vi "change CAD coordinates.vi"() -> ()   [LabVIEW 2020]
uses:
  <vilib>/Analysis/NI_AALPro.lvlib
  <vilib>/Analysis/coordinate.llb/2D Cartesian Coordinate Rotation (Scalar).vi
panel:
  in  "Save to txt file":bool
  in  "Save picture":bool
  out "2D Picture":picture
  in  "Add delamination dots":bool
  out "Array":dbl[][](array[numeric])
  in  "stop":bool
  in  "Rotate by angle":bool
  in  "theta (degrees)":dbl
  in  "Flip Y sign":bool
  in  "Flip X sign":bool
  in  "increase radius":bool
  in  "inc":dbl format="%#_13g"
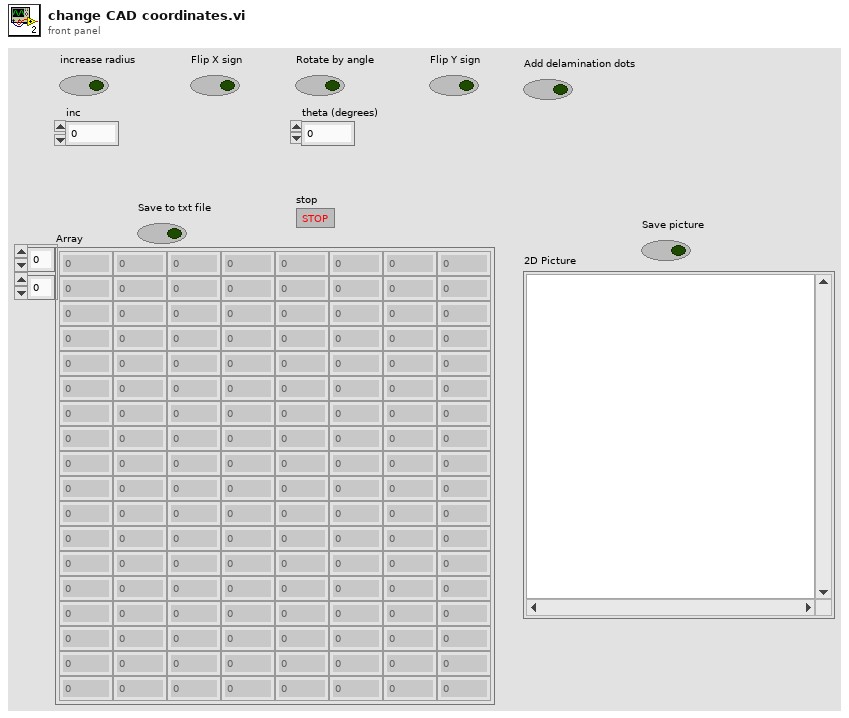
[diagram p1: front panel]
types:
  T1 = typedef "imagedata.ctl" = cluster{"image type":i32, "image depth":i32, "image":u8[], "mask":u8[], "colors":u32[], "Rectangle":cluster{"left":i16, "top":i16, "right":i16, "bottom":i16}}
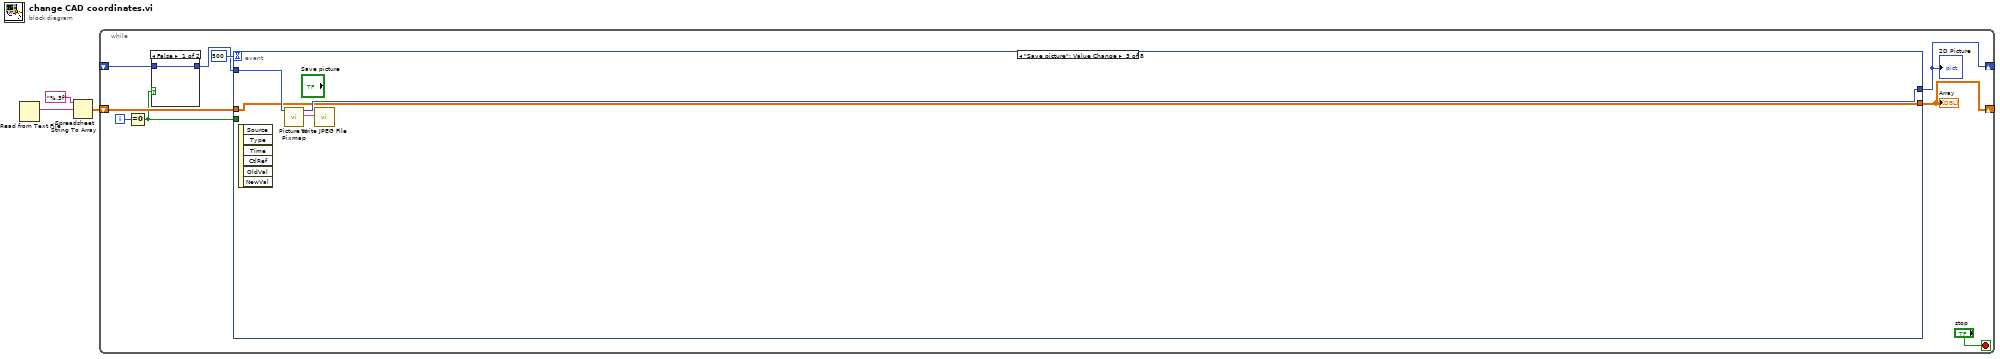
[diagram p0: block diagram]
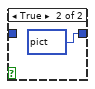
[diagram p2: hidden frame]
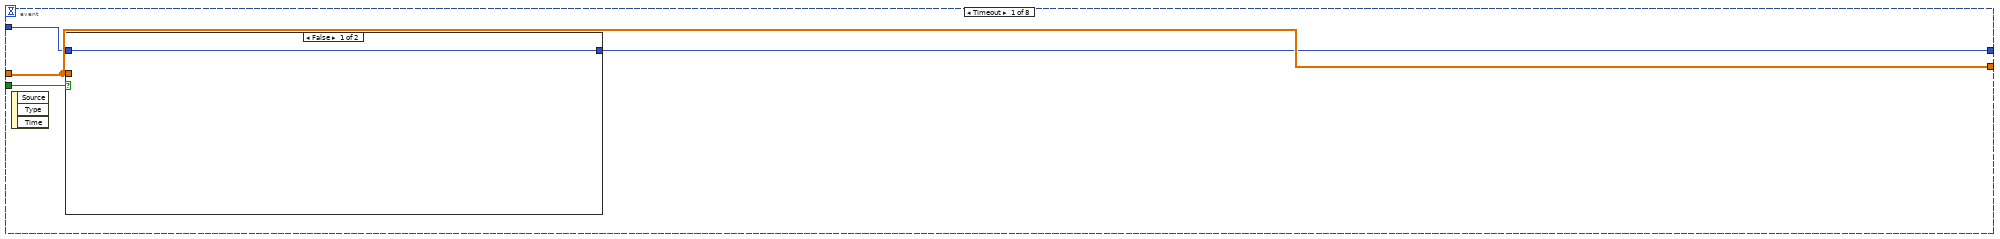
[diagram p3: hidden frame]
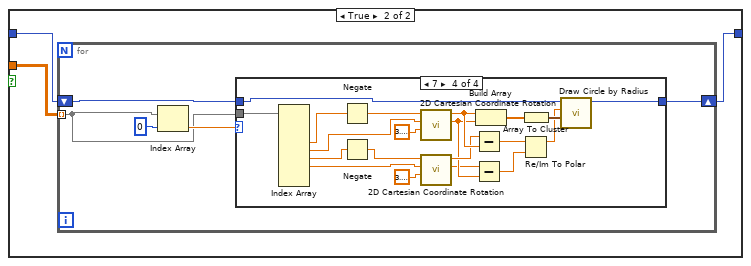
[diagram p4: hidden frame]
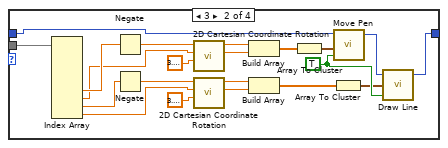
[diagram p6: hidden frame]
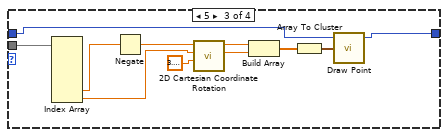
[diagram p7: hidden frame]
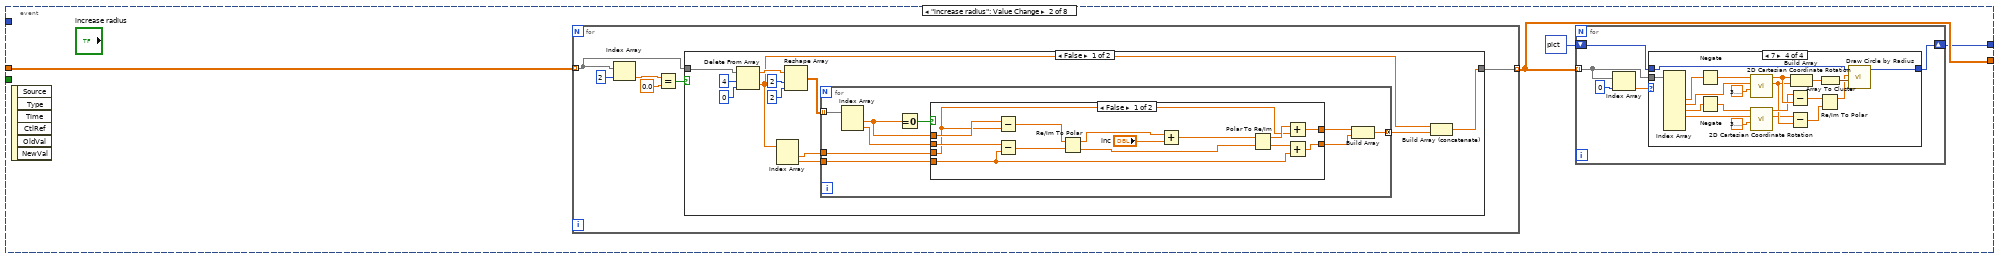
[diagram p8: hidden frame]
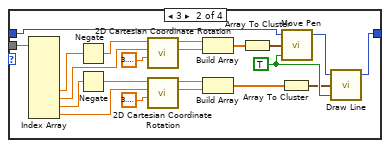
[diagram p10: hidden frame]
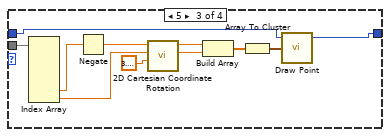
[diagram p11: hidden frame]
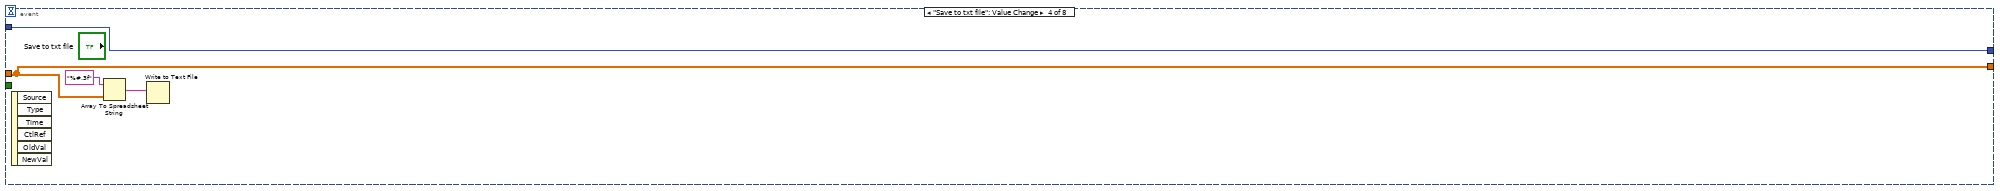
[diagram p14: hidden frame]
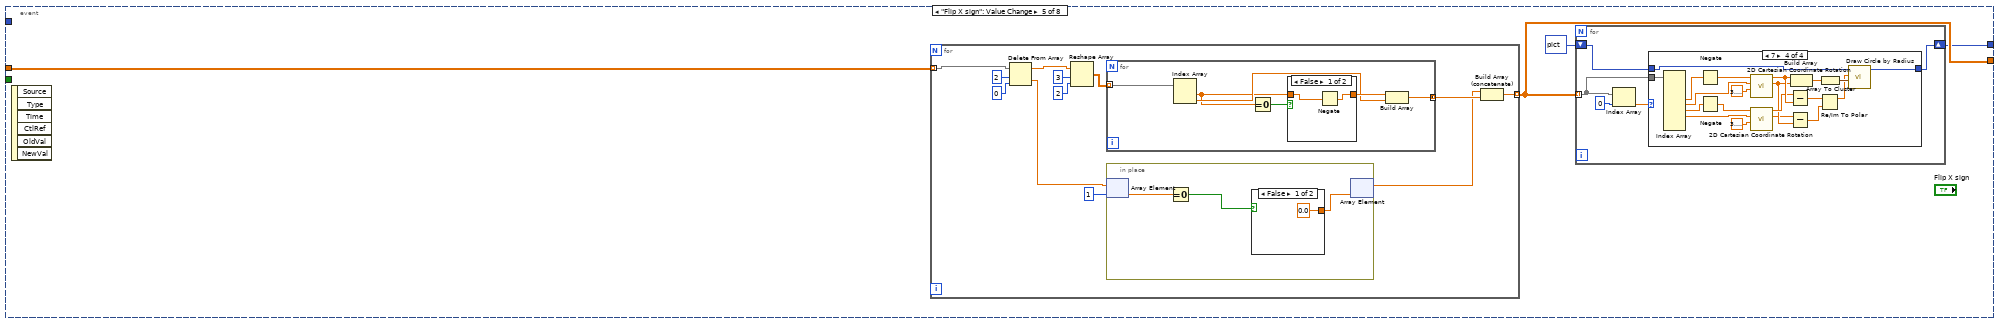
[diagram p15: hidden frame]
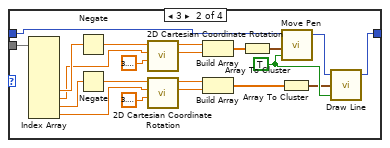
[diagram p17: hidden frame]
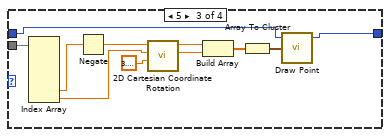
[diagram p18: hidden frame]
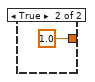
[diagram p19: hidden frame]
diagram:
  n1 = Read from Text File() -> (text=w3:string)  [unwired: 4 in, 3 out]
  n2 = Spreadsheet String To Array(format string="%.3f", spreadsheet string=w3) -> (array=w1:dbl[][])  [unwired: 2 in]
  n3 = while {
    shift-right: [w4] -> _
    shift-left: w1 -> [w10]
    shift-right: [w5] -> _
    shift-left: _ -> [w6]
    i -> [w9]
    stop <- "stop" stop-if-true
    n4 = Equal To 0?(x=w9) -> (x = 0?=w8:bool)
    n5 = case shown="False" w8 {
      tunnel: [w13 picture data[5B] ("picture")] -> w7
      tunnel: w6 -> [w13 _]
      frame False {
      }
      frame True {
      }
    }
    n6 = event shown="[2] \"Save picture\": Value Change" {
      selector: _ -> [_ _ _ _ _ _ _ _]
      dyn-events: _ -> [_ _ _ _ _ _ _ _]
      timeout: 500 -> [_ _ _ _ _ _ _ _]
      tunnel: w10 -> [w18 w84 w187 w192 w198 w286 w367 w482]
      tunnel: [w18 w83 w187 w192 w197 w285 w366 w473] -> w4
      tunnel: [w17 w82 w188 w191 w196 w284 w365 w472] -> w5
      tunnel: w7 -> [w16 _ w189 w191 _ _ _ _]
      tunnel: w8 -> [w15 _ _ _ _ _ _ _]
      event Timeout {
        n7 = event-data() -> ()  [unwired: 1 in, 3 out]
        n8 = case shown="False" w15 {
          tunnel: w16 -> [w19 w22]
          tunnel: w18 -> [_ w21]
          tunnel: [w19 w20] -> w17
          frame False {
          }
          frame True {
            n9 = for {
              tunnel: w21 -> [w25] mode=indexing
              shift-right: [w23] -> w20
              shift-left: w22 -> [w24]
              n10 = Index Array(array=w25, index=0) -> (element=w26:dbl)
              n11 = case shown="7" w26 {
                tunnel: w25 -> [_ w45 w58 w76]
                tunnel: w24 -> [w28 w47 w60 w80]
                tunnel: [w28 w49 w59 w79] -> w23
                frame 0, Default {
                }
                frame 3 {
                  w46 = TRUE ("absolute coordinates?(T)")
                  n12 = Index Array(array=w45) -> (element #5=w40:dbl, element #6=w37:dbl, element #7=w39:dbl, element #8=w31:dbl)  [unwired: 8 in, 4 out]
                  n13 = Negate(x=w40) -> (-x=w38:dbl)
                  n14 = Negate(x=w39) -> (-x=w32:dbl)
                  n15 = call-poly <vilib>:"2D Cartesian Coordinate Rotation.vi"("theta"=3.141592653589793, "y"=w37, "x"=w38) -> ("y out"=w34:dbl, "x out"=w35:dbl)  [unwired: 6 in, 1 out]
                  n16 = call-poly <vilib>:"2D Cartesian Coordinate Rotation.vi"("theta"=3.141592653589793, "y"=w31, "x"=w32) -> ("y out"=w29:dbl, "x out"=w30:dbl)  [unwired: 6 in, 1 out]
                  n17 = Build Array(w35, w34) -> (w44:dbl[])
                  n18 = Build Array(w30, w29) -> (w42:dbl[])
                  n19 = Array To Cluster(array=w44) -> (cluster=w43:cluster{"[0]":dbl, "[1]":dbl})
                  n20 = Array To Cluster(array=w42) -> (cluster=w41:cluster{"[0]":dbl, "[1]":dbl})
                  n21 = call <vilib>:"Move Pen.vi"("absolute coordinates?(T)"=w46, "new position"=w43, "picture"=w47) -> ("new picture"=w48:picture)  [unwired: 2 in]
                  n22 = call <vilib>:"Draw Line.vi"("picture"=w48, "end point"=w41, "absolute coordinates?(T)"=w46) -> ("new picture"=w49:picture)  [unwired: 6 in]
                }
                frame 5 {
                  n23 = Index Array(array=w58) -> (element #5=w55:dbl, element #6=w52:dbl)  [unwired: 6 in, 4 out]
                  n24 = Negate(x=w55) -> (-x=w53:dbl)
                  n25 = call-poly <vilib>:"2D Cartesian Coordinate Rotation.vi"("theta"=3.141592653589793, "y"=w52, "x"=w53) -> ("y out"=w50:dbl, "x out"=w51:dbl)  [unwired: 6 in, 1 out]
                  n26 = Build Array(w51, w50) -> (w57:dbl[])
                  n27 = Array To Cluster(array=w57) -> (cluster=w56:cluster{"[0]":dbl, "[1]":dbl})
                  n28 = call <vilib>:"Draw Point.vi"("picture"=w60, "point(x,y)"=w56) -> ("new picture"=w59:picture)  [unwired: 7 in]
                }
                frame 7 {
                  n29 = Index Array(array=w76) -> (element #3=w73:dbl, element #4=w68:dbl, element #5=w72:dbl, element #6=w63:dbl)  [unwired: 8 in, 4 out]
                  n30 = Negate(x=w73) -> (-x=w69:dbl)
                  n31 = Negate(x=w72) -> (-x=w66:dbl)
                  n32 = call-poly <vilib>:"2D Cartesian Coordinate Rotation.vi"("theta"=3.141592653589793, "y"=w68, "x"=w69) -> ("y out"=w64:dbl, "x out"=w70:dbl)  [unwired: 6 in, 1 out]
                  n33 = call-poly <vilib>:"2D Cartesian Coordinate Rotation.vi"("theta"=3.141592653589793, "y"=w63, "x"=w66) -> ("y out"=w62:dbl, "x out"=w65:dbl)  [unwired: 6 in, 1 out]
                  n34 = Subtract(x=w65, y=w70) -> (x-y=w75:dbl)
                  n35 = Subtract(x=w62, y=w64) -> (x-y=w61:dbl)
                  n36 = Build Array(w70, w64) -> (w78:dbl[])
                  n37 = Array To Cluster(array=w78) -> (cluster=w77:cluster{"[0]":dbl, "[1]":dbl})
                  n38 = Re/Im To Polar(2:w61, 3:w75) -> (1:w74:dbl)  [unwired: 1 out]
                  n39 = call <vilib>:"Draw Circle by Radius.vi"("pixel center"=w77, "radius"=w74, "picture"=w80) -> ("new picture"=w79:picture)  [unwired: 8 in]
                }
              }
            }
          }
        }
      }
      event "increase radius": Value Change {
        n40 = event-data() -> ()  [unwired: 1 in, 6 out]
        n41 = for {
          tunnel: [w146] -> w83 mode=indexing
          tunnel: w84 -> [w145] mode=indexing
          n42 = Index Array(array=w145, index=2) -> (element=w143:dbl)
          n43 = Equal?(x=w143, y=0.0) -> (x = y?=w147:bool)
          n44 = case shown="False" w147 {
            tunnel: [w149 w186] -> w146
            tunnel: w145 -> [w155 w186]
            frame False {
              n45 = Delete From Array(array=w155, length=4, index=0) -> (deleted portion=w154:dbl[], array with subset deleted=w156:dbl[])
              n46 = Index Array(array=w154) -> (element #1=w152:dbl, element #2=w151:dbl)  [unwired: 2 in]
              n47 = Reshape Array(w156, 2 ("dimension size"), 2 ("dimension size")) -> (w153:dbl[][])
              n48 = for {
                tunnel: w153 -> [w169] mode=indexing
                tunnel: w152 -> [w167]
                tunnel: w151 -> [w163]
                tunnel: [w164] -> w150 mode=concatenating
                n49 = Index Array(array=w169) -> (element #1=w161:dbl, element #2=w168:dbl)  [unwired: 2 in]
                n50 = Equal To 0?(x=w161) -> (x = 0?=w162:bool)
                n51 = case shown="False" w162 {
                  tunnel: w161 -> [w183 w185]
                  tunnel: w168 -> [w181 w184]
                  tunnel: w167 -> [w174 _]
                  tunnel: [w173 w185] -> w166
                  tunnel: w163 -> [w171 _]
                  tunnel: [w170 w184] -> w165
                  frame False {
                    n52 = Subtract(x=w183, y=w174) -> (x-y=w182:dbl)
                    n53 = Subtract(x=w181, y=w171) -> (x-y=w180:dbl)
                    n54 = Re/Im To Polar(2:w180, 3:w182) -> (0:w177:dbl, 1:w179:dbl)
                    n55 = Add(x=w179, y="inc") -> (x+y=w176:dbl)
                    n56 = Polar To Re/Im(2:w177, 3:w176) -> (0:w172:dbl, 1:w175:dbl)
                    n57 = Add(x=w175, y=w174) -> (x+y=w173:dbl)
                    n58 = Add(x=w172, y=w171) -> (x+y=w170:dbl)
                  }
                  frame True {
                  }
                }
                n59 = Build Array(w166, w165) -> (w164:dbl[])
              }
              n60 = Build Array (concatenate)(w154, w150) -> (w149:dbl[])
            }
            frame True {
            }
          }
        }
        n61 = for {
          tunnel: w83 -> [w87] mode=indexing
          shift-right: [w85] -> w82
          shift-left: picture data[5B] ("new picture") -> [w86]
          n62 = Index Array(array=w87, index=0) -> (element=w88:dbl)
          n63 = case shown="7" w88 {
            tunnel: w87 -> [_ w107 w120 w138]
            tunnel: w86 -> [w90 w109 w122 w142]
            tunnel: [w90 w111 w121 w141] -> w85
            frame 0, Default {
            }
            frame 3 {
              w108 = TRUE ("absolute coordinates?(T)")
              n64 = Index Array(array=w107) -> (element #5=w102:dbl, element #6=w99:dbl, element #7=w101:dbl, element #8=w93:dbl)  [unwired: 8 in, 4 out]
              n65 = Negate(x=w102) -> (-x=w100:dbl)
              n66 = Negate(x=w101) -> (-x=w94:dbl)
              n67 = call-poly <vilib>:"2D Cartesian Coordinate Rotation.vi"("theta"=3.141592653589793, "y"=w99, "x"=w100) -> ("y out"=w96:dbl, "x out"=w97:dbl)  [unwired: 6 in, 1 out]
              n68 = call-poly <vilib>:"2D Cartesian Coordinate Rotation.vi"("theta"=3.141592653589793, "y"=w93, "x"=w94) -> ("y out"=w91:dbl, "x out"=w92:dbl)  [unwired: 6 in, 1 out]
              n69 = Build Array(w97, w96) -> (w106:dbl[])
              n70 = Build Array(w92, w91) -> (w104:dbl[])
              n71 = Array To Cluster(array=w106) -> (cluster=w105:cluster{"[0]":dbl, "[1]":dbl})
              n72 = Array To Cluster(array=w104) -> (cluster=w103:cluster{"[0]":dbl, "[1]":dbl})
              n73 = call <vilib>:"Move Pen.vi"("absolute coordinates?(T)"=w108, "new position"=w105, "picture"=w109) -> ("new picture"=w110:picture)  [unwired: 2 in]
              n74 = call <vilib>:"Draw Line.vi"("picture"=w110, "end point"=w103, "absolute coordinates?(T)"=w108) -> ("new picture"=w111:picture)  [unwired: 6 in]
            }
            frame 5 {
              n75 = Index Array(array=w120) -> (element #5=w117:dbl, element #6=w114:dbl)  [unwired: 6 in, 4 out]
              n76 = Negate(x=w117) -> (-x=w115:dbl)
              n77 = call-poly <vilib>:"2D Cartesian Coordinate Rotation.vi"("theta"=3.141592653589793, "y"=w114, "x"=w115) -> ("y out"=w112:dbl, "x out"=w113:dbl)  [unwired: 6 in, 1 out]
              n78 = Build Array(w113, w112) -> (w119:dbl[])
              n79 = Array To Cluster(array=w119) -> (cluster=w118:cluster{"[0]":dbl, "[1]":dbl})
              n80 = call <vilib>:"Draw Point.vi"("picture"=w122, "point(x,y)"=w118) -> ("new picture"=w121:picture)  [unwired: 7 in]
            }
            frame 7 {
              n81 = Index Array(array=w138) -> (element #3=w135:dbl, element #4=w130:dbl, element #5=w134:dbl, element #6=w125:dbl)  [unwired: 8 in, 4 out]
              n82 = Negate(x=w135) -> (-x=w131:dbl)
              n83 = Negate(x=w134) -> (-x=w128:dbl)
              n84 = call-poly <vilib>:"2D Cartesian Coordinate Rotation.vi"("theta"=3.141592653589793, "y"=w130, "x"=w131) -> ("y out"=w126:dbl, "x out"=w132:dbl)  [unwired: 6 in, 1 out]
              n85 = call-poly <vilib>:"2D Cartesian Coordinate Rotation.vi"("theta"=3.141592653589793, "y"=w125, "x"=w128) -> ("y out"=w124:dbl, "x out"=w127:dbl)  [unwired: 6 in, 1 out]
              n86 = Subtract(x=w127, y=w132) -> (x-y=w137:dbl)
              n87 = Subtract(x=w124, y=w126) -> (x-y=w123:dbl)
              n88 = Build Array(w132, w126) -> (w140:dbl[])
              n89 = Array To Cluster(array=w140) -> (cluster=w139:cluster{"[0]":dbl, "[1]":dbl})
              n90 = Re/Im To Polar(2:w123, 3:w137) -> (1:w136:dbl)  [unwired: 1 out]
              n91 = call <vilib>:"Draw Circle by Radius.vi"("pixel center"=w139, "radius"=w136, "picture"=w142) -> ("new picture"=w141:picture)  [unwired: 8 in]
            }
          }
        }
      }
      event "Save picture": Value Change {
        n92 = event-data() -> ()  [unwired: 1 in, 6 out]
        n93 = call <vilib>:"Picture to Pixmap.vi"("picture"=w189) -> ("image data"=w190:T1, "new picture"=w188:picture)  [unwired: 9 in]
        n94 = call <vilib>:"Write JPEG File.vi"("image data"=w190) -> ()  [unwired: 9 in, 2 out]
      }
      event "Save to txt file": Value Change {
        n95 = event-data() -> ()  [unwired: 1 in, 6 out]
        n96 = Array To Spreadsheet String(array=w192, 3:"%#.3f" ("format string")) -> (spreadsheet string=w194:string)  [unwired: 1 in]
        n97 = Write to Text File(text=w194) -> ()  [unwired: 3 in, 3 out]
      }
      event "Flip X sign": Value Change {
        n98 = event-data() -> ()  [unwired: 1 in, 6 out]
        n99 = for {
          tunnel: w198 -> [w267] mode=indexing
          tunnel: [w268] -> w197 mode=indexing
          n100 = Delete From Array(array=w267, length=2, index=0) -> (deleted portion=w259:dbl[], array with subset deleted=w262:dbl[])
          n101 = Reshape Array(w262, 3 ("dimension size"), 2 ("dimension size")) -> (w261:dbl[][])
          n102 = for {
            tunnel: w261 -> [w279] mode=indexing
            tunnel: [w276] -> w260 mode=concatenating
            n103 = Index Array(array=w279) -> (element #1=w274:dbl, element #2=w277:dbl)  [unwired: 2 in]
            n104 = Equal To 0?(x=w274) -> (x = 0?=w275:bool)
            n105 = case shown="False" w275 {
              tunnel: w274 -> [w281 w282]
              tunnel: [w280 w282] -> w278
              frame False {
                n106 = Negate(x=w281) -> (-x=w280:dbl)
              }
              frame True {
              }
            }
            n107 = Build Array(w278, w277) -> (w276:dbl[])
          }
          n108 = in-place {
            n109 = in-place-array #1(w259, 1) -> (w270:dbl)
            n110 = Equal To 0?(x=w270) -> (x = 0?=w271:bool)
            n111 = case shown="False" w271 {
              tunnel: [0.0 1.0] -> w269
              frame False {
              }
              frame True {
              }
            }
            n112 = in-place-array #1(w269) -> (w258:dbl[])  [unwired: 1 out]
          }
          n113 = Build Array (concatenate)(w258, w260) -> (w268:dbl[])
        }
        n114 = for {
          tunnel: w197 -> [w201] mode=indexing
          shift-right: [w199] -> w196
          shift-left: picture data[5B] ("new picture") -> [w200]
          n115 = Index Array(array=w201, index=0) -> (element=w202:dbl)
          n116 = case shown="7" w202 {
            tunnel: w201 -> [_ w221 w234 w252]
            tunnel: w200 -> [w204 w223 w236 w256]
            tunnel: [w204 w225 w235 w255] -> w199
            frame 0, Default {
            }
            frame 3 {
              w222 = TRUE ("absolute coordinates?(T)")
              n117 = Index Array(array=w221) -> (element #5=w216:dbl, element #6=w213:dbl, element #7=w215:dbl, element #8=w207:dbl)  [unwired: 8 in, 4 out]
              n118 = Negate(x=w216) -> (-x=w214:dbl)
              n119 = Negate(x=w215) -> (-x=w208:dbl)
              n120 = call-poly <vilib>:"2D Cartesian Coordinate Rotation.vi"("theta"=3.141592653589793, "y"=w213, "x"=w214) -> ("y out"=w210:dbl, "x out"=w211:dbl)  [unwired: 6 in, 1 out]
              n121 = call-poly <vilib>:"2D Cartesian Coordinate Rotation.vi"("theta"=3.141592653589793, "y"=w207, "x"=w208) -> ("y out"=w205:dbl, "x out"=w206:dbl)  [unwired: 6 in, 1 out]
              n122 = Build Array(w211, w210) -> (w220:dbl[])
              n123 = Build Array(w206, w205) -> (w218:dbl[])
              n124 = Array To Cluster(array=w220) -> (cluster=w219:cluster{"[0]":dbl, "[1]":dbl})
              n125 = Array To Cluster(array=w218) -> (cluster=w217:cluster{"[0]":dbl, "[1]":dbl})
              n126 = call <vilib>:"Move Pen.vi"("absolute coordinates?(T)"=w222, "new position"=w219, "picture"=w223) -> ("new picture"=w224:picture)  [unwired: 2 in]
              n127 = call <vilib>:"Draw Line.vi"("picture"=w224, "end point"=w217, "absolute coordinates?(T)"=w222) -> ("new picture"=w225:picture)  [unwired: 6 in]
            }
            frame 5 {
              n128 = Index Array(array=w234) -> (element #5=w231:dbl, element #6=w228:dbl)  [unwired: 6 in, 4 out]
              n129 = Negate(x=w231) -> (-x=w229:dbl)
              n130 = call-poly <vilib>:"2D Cartesian Coordinate Rotation.vi"("theta"=3.141592653589793, "y"=w228, "x"=w229) -> ("y out"=w226:dbl, "x out"=w227:dbl)  [unwired: 6 in, 1 out]
              n131 = Build Array(w227, w226) -> (w233:dbl[])
              n132 = Array To Cluster(array=w233) -> (cluster=w232:cluster{"[0]":dbl, "[1]":dbl})
              n133 = call <vilib>:"Draw Point.vi"("picture"=w236, "point(x,y)"=w232) -> ("new picture"=w235:picture)  [unwired: 7 in]
            }
            frame 7 {
              n134 = Index Array(array=w252) -> (element #3=w249:dbl, element #4=w244:dbl, element #5=w248:dbl, element #6=w239:dbl)  [unwired: 8 in, 4 out]
              n135 = Negate(x=w249) -> (-x=w245:dbl)
              n136 = Negate(x=w248) -> (-x=w242:dbl)
              n137 = call-poly <vilib>:"2D Cartesian Coordinate Rotation.vi"("theta"=3.141592653589793, "y"=w244, "x"=w245) -> ("y out"=w240:dbl, "x out"=w246:dbl)  [unwired: 6 in, 1 out]
              n138 = call-poly <vilib>:"2D Cartesian Coordinate Rotation.vi"("theta"=3.141592653589793, "y"=w239, "x"=w242) -> ("y out"=w238:dbl, "x out"=w241:dbl)  [unwired: 6 in, 1 out]
              n139 = Subtract(x=w241, y=w246) -> (x-y=w251:dbl)
              n140 = Subtract(x=w238, y=w240) -> (x-y=w237:dbl)
              n141 = Build Array(w246, w240) -> (w254:dbl[])
              n142 = Array To Cluster(array=w254) -> (cluster=w253:cluster{"[0]":dbl, "[1]":dbl})
              n143 = Re/Im To Polar(2:w237, 3:w251) -> (1:w250:dbl)  [unwired: 1 out]
              n144 = call <vilib>:"Draw Circle by Radius.vi"("pixel center"=w253, "radius"=w250, "picture"=w256) -> ("new picture"=w255:picture)  [unwired: 8 in]
            }
          }
        }
      }
      event "Flip Y sign": Value Change {
        n145 = event-data() -> ()  [unwired: 1 in, 6 out]
        n146 = for {
          tunnel: w286 -> [w353] mode=indexing
          tunnel: [w354] -> w285 mode=indexing
          n147 = Delete From Array(array=w353, length=2, index=0) -> (deleted portion=w346:dbl[], array with subset deleted=w348:dbl[])
          n148 = Reshape Array(w348, 3 ("dimension size"), 2 ("dimension size")) -> (w347:dbl[][])
          n149 = for {
            tunnel: w347 -> [w360] mode=indexing
            tunnel: [w359] -> w345 mode=concatenating
            n150 = Index Array(array=w360) -> (element #1=w356:dbl, element #2=w357:dbl)  [unwired: 2 in]
            n151 = Equal To 0?(x=w357) -> (x = 0?=w358:bool)
            n152 = case shown="False" w358 {
              tunnel: [w362 w363] -> w355
              tunnel: w357 -> [w361 w363]
              frame False {
                n153 = Negate(x=w361) -> (-x=w362:dbl)
              }
              frame True {
              }
            }
            n154 = Build Array(w356, w355) -> (w359:dbl[])
          }
          n155 = Build Array (concatenate)(w346, w345) -> (w354:dbl[])
        }
        n156 = for {
          tunnel: w285 -> [w289] mode=indexing
          shift-right: [w287] -> w284
          shift-left: picture data[5B] ("new picture") -> [w288]
          n157 = Index Array(array=w289, index=0) -> (element=w290:dbl)
          n158 = case shown="7" w290 {
            tunnel: w289 -> [_ w309 w322 w340]
            tunnel: w288 -> [w292 w311 w324 w344]
            tunnel: [w292 w313 w323 w343] -> w287
            frame 0, Default {
            }
            frame 3 {
              w310 = TRUE ("absolute coordinates?(T)")
              n159 = Index Array(array=w309) -> (element #5=w304:dbl, element #6=w301:dbl, element #7=w303:dbl, element #8=w295:dbl)  [unwired: 8 in, 4 out]
              n160 = Negate(x=w304) -> (-x=w302:dbl)
              n161 = Negate(x=w303) -> (-x=w296:dbl)
              n162 = call-poly <vilib>:"2D Cartesian Coordinate Rotation.vi"("theta"=3.141592653589793, "y"=w301, "x"=w302) -> ("y out"=w298:dbl, "x out"=w299:dbl)  [unwired: 6 in, 1 out]
              n163 = call-poly <vilib>:"2D Cartesian Coordinate Rotation.vi"("theta"=3.141592653589793, "y"=w295, "x"=w296) -> ("y out"=w293:dbl, "x out"=w294:dbl)  [unwired: 6 in, 1 out]
              n164 = Build Array(w299, w298) -> (w308:dbl[])
              n165 = Build Array(w294, w293) -> (w306:dbl[])
              n166 = Array To Cluster(array=w308) -> (cluster=w307:cluster{"[0]":dbl, "[1]":dbl})
              n167 = Array To Cluster(array=w306) -> (cluster=w305:cluster{"[0]":dbl, "[1]":dbl})
              n168 = call <vilib>:"Move Pen.vi"("absolute coordinates?(T)"=w310, "new position"=w307, "picture"=w311) -> ("new picture"=w312:picture)  [unwired: 2 in]
              n169 = call <vilib>:"Draw Line.vi"("picture"=w312, "end point"=w305, "absolute coordinates?(T)"=w310) -> ("new picture"=w313:picture)  [unwired: 6 in]
            }
            frame 5 {
              n170 = Index Array(array=w322) -> (element #5=w319:dbl, element #6=w316:dbl)  [unwired: 6 in, 4 out]
              n171 = Negate(x=w319) -> (-x=w317:dbl)
              n172 = call-poly <vilib>:"2D Cartesian Coordinate Rotation.vi"("theta"=3.141592653589793, "y"=w316, "x"=w317) -> ("y out"=w314:dbl, "x out"=w315:dbl)  [unwired: 6 in, 1 out]
              n173 = Build Array(w315, w314) -> (w321:dbl[])
              n174 = Array To Cluster(array=w321) -> (cluster=w320:cluster{"[0]":dbl, "[1]":dbl})
              n175 = call <vilib>:"Draw Point.vi"("picture"=w324, "point(x,y)"=w320) -> ("new picture"=w323:picture)  [unwired: 7 in]
            }
            frame 7 {
              n176 = Index Array(array=w340) -> (element #3=w337:dbl, element #4=w332:dbl, element #5=w336:dbl, element #6=w327:dbl)  [unwired: 8 in, 4 out]
              n177 = Negate(x=w337) -> (-x=w333:dbl)
              n178 = Negate(x=w336) -> (-x=w330:dbl)
              n179 = call-poly <vilib>:"2D Cartesian Coordinate Rotation.vi"("theta"=3.141592653589793, "y"=w332, "x"=w333) -> ("y out"=w328:dbl, "x out"=w334:dbl)  [unwired: 6 in, 1 out]
              n180 = call-poly <vilib>:"2D Cartesian Coordinate Rotation.vi"("theta"=3.141592653589793, "y"=w327, "x"=w330) -> ("y out"=w326:dbl, "x out"=w329:dbl)  [unwired: 6 in, 1 out]
              n181 = Subtract(x=w329, y=w334) -> (x-y=w339:dbl)
              n182 = Subtract(x=w326, y=w328) -> (x-y=w325:dbl)
              n183 = Build Array(w334, w328) -> (w342:dbl[])
              n184 = Array To Cluster(array=w342) -> (cluster=w341:cluster{"[0]":dbl, "[1]":dbl})
              n185 = Re/Im To Polar(2:w325, 3:w339) -> (1:w338:dbl)  [unwired: 1 out]
              n186 = call <vilib>:"Draw Circle by Radius.vi"("pixel center"=w341, "radius"=w338, "picture"=w344) -> ("new picture"=w343:picture)  [unwired: 8 in]
            }
          }
        }
      }
      event "Rotate by angle": Value Change {
        n187 = event-data() -> ()  [unwired: 1 in, 6 out]
        n188 = for {
          tunnel: w367 -> [w435] mode=indexing
          tunnel: [w434] -> w366 mode=indexing
          n189 = in-place {
            n190 = in-place-array #2(w435, 0, 1, 2, 3, 4, 5, 6, 7) -> (w449:dbl, w448:dbl, w447:dbl, w444:dbl, w443:dbl, w440:dbl, w439:dbl, w436:dbl)
            n191 = Equal To 0?(x=w449) -> (x = 0?=w450:bool)
            n192 = case shown="False" w450 {
              tunnel: [w461 w470] -> w446
              tunnel: w447 -> [w464 w470]
              tunnel: w444 -> [w463 w469]
              tunnel: [w460 w469] -> w445
              tunnel: w443 -> [w459 w468]
              tunnel: [w457 w468] -> w442
              tunnel: [w456 w467] -> w441
              tunnel: w440 -> [w458 w467]
              tunnel: w439 -> [w453 w466]
              tunnel: [w455 w466] -> w438
              tunnel: [w454 w465] -> w437
              tunnel: w436 -> [w452 w465]
              frame False {
                n193 = expression code="(x/180.0)*pi" "degrees to radians"("theta (degrees)") -> (w451:dbl)
                n194 = call-poly <vilib>:"2D Cartesian Coordinate Rotation.vi"("theta"=w451, "y"=w463, "x"=w464) -> ("y out"=w460:dbl, "x out"=w461:dbl)  [unwired: 6 in, 1 out]
                n195 = call-poly <vilib>:"2D Cartesian Coordinate Rotation.vi"("theta"=w451, "y"=w458, "x"=w459) -> ("y out"=w456:dbl, "x out"=w457:dbl)  [unwired: 6 in, 1 out]
                n196 = call-poly <vilib>:"2D Cartesian Coordinate Rotation.vi"("theta"=w451, "y"=w452, "x"=w453) -> ("y out"=w454:dbl, "x out"=w455:dbl)  [unwired: 6 in, 1 out]
              }
              frame True {
              }
            }
            n197 = in-place-array #2(w449, w448, w446, w445, w442, w441, w438, w437) -> (w434:dbl[])  [unwired: 8 out]
          }
        }
        n198 = for {
          tunnel: w366 -> [w370] mode=indexing
          shift-right: [w368] -> w365
          shift-left: picture data[5B] ("new picture") -> [w369]
          n199 = Index Array(array=w370, index=0) -> (element=w371:dbl)
          n200 = case shown="7" w371 {
            tunnel: w370 -> [_ w390 w403 w421]
            tunnel: w369 -> [w373 w392 w405 w425]
            tunnel: [w373 w394 w404 w424] -> w368
            frame 0, Default {
            }
            frame 3 {
              w391 = TRUE ("absolute coordinates?(T)")
              n201 = Index Array(array=w390) -> (element #5=w385:dbl, element #6=w382:dbl, element #7=w384:dbl, element #8=w376:dbl)  [unwired: 8 in, 4 out]
              n202 = Negate(x=w385) -> (-x=w383:dbl)
              n203 = Negate(x=w384) -> (-x=w377:dbl)
              n204 = call-poly <vilib>:"2D Cartesian Coordinate Rotation.vi"("theta"=3.141592653589793, "y"=w382, "x"=w383) -> ("y out"=w379:dbl, "x out"=w380:dbl)  [unwired: 6 in, 1 out]
              n205 = call-poly <vilib>:"2D Cartesian Coordinate Rotation.vi"("theta"=3.141592653589793, "y"=w376, "x"=w377) -> ("y out"=w374:dbl, "x out"=w375:dbl)  [unwired: 6 in, 1 out]
              n206 = Build Array(w380, w379) -> (w389:dbl[])
              n207 = Build Array(w375, w374) -> (w387:dbl[])
              n208 = Array To Cluster(array=w389) -> (cluster=w388:cluster{"[0]":dbl, "[1]":dbl})
              n209 = Array To Cluster(array=w387) -> (cluster=w386:cluster{"[0]":dbl, "[1]":dbl})
              n210 = call <vilib>:"Move Pen.vi"("absolute coordinates?(T)"=w391, "new position"=w388, "picture"=w392) -> ("new picture"=w393:picture)  [unwired: 2 in]
              n211 = call <vilib>:"Draw Line.vi"("picture"=w393, "end point"=w386, "absolute coordinates?(T)"=w391) -> ("new picture"=w394:picture)  [unwired: 6 in]
            }
            frame 5 {
              n212 = Index Array(array=w403) -> (element #5=w400:dbl, element #6=w397:dbl)  [unwired: 6 in, 4 out]
              n213 = Negate(x=w400) -> (-x=w398:dbl)
              n214 = call-poly <vilib>:"2D Cartesian Coordinate Rotation.vi"("theta"=3.141592653589793, "y"=w397, "x"=w398) -> ("y out"=w395:dbl, "x out"=w396:dbl)  [unwired: 6 in, 1 out]
              n215 = Build Array(w396, w395) -> (w402:dbl[])
              n216 = Array To Cluster(array=w402) -> (cluster=w401:cluster{"[0]":dbl, "[1]":dbl})
              n217 = call <vilib>:"Draw Point.vi"("picture"=w405, "point(x,y)"=w401) -> ("new picture"=w404:picture)  [unwired: 7 in]
            }
            frame 7 {
              n218 = Index Array(array=w421) -> (element #3=w418:dbl, element #4=w413:dbl, element #5=w417:dbl, element #6=w408:dbl)  [unwired: 8 in, 4 out]
              n219 = Negate(x=w418) -> (-x=w414:dbl)
              n220 = Negate(x=w417) -> (-x=w411:dbl)
              n221 = call-poly <vilib>:"2D Cartesian Coordinate Rotation.vi"("theta"=3.141592653589793, "y"=w413, "x"=w414) -> ("y out"=w409:dbl, "x out"=w415:dbl)  [unwired: 6 in, 1 out]
              n222 = call-poly <vilib>:"2D Cartesian Coordinate Rotation.vi"("theta"=3.141592653589793, "y"=w408, "x"=w411) -> ("y out"=w407:dbl, "x out"=w410:dbl)  [unwired: 6 in, 1 out]
              n223 = Subtract(x=w410, y=w415) -> (x-y=w420:dbl)
              n224 = Subtract(x=w407, y=w409) -> (x-y=w406:dbl)
              n225 = Build Array(w415, w409) -> (w423:dbl[])
              n226 = Array To Cluster(array=w423) -> (cluster=w422:cluster{"[0]":dbl, "[1]":dbl})
              n227 = Re/Im To Polar(2:w406, 3:w420) -> (1:w419:dbl)  [unwired: 1 out]
              n228 = call <vilib>:"Draw Circle by Radius.vi"("pixel center"=w422, "radius"=w419, "picture"=w425) -> ("new picture"=w424:picture)  [unwired: 8 in]
            }
          }
        }
      }
      event "Add delamination dots": Value Change {
        n229 = event-data() -> ()  [unwired: 1 in, 6 out]
        n230 = for {
          N: 6 -> [_]
          shift-right: [w604] -> _
          shift-left: 0.0 ("theta") -> [w600]
          tunnel: [w603] -> w479 mode=indexing
          n231 = expression code="(x/180.0)*pi" "degrees to radians"(w600) -> (w606:dbl)
          n232 = call-poly <vilib>:"2D Cartesian Coordinate Rotation.vi"("theta"=w606, "y"=0.0, "x"=15.0) -> ("y out"=w601:dbl, "x out"=w602:dbl)  [unwired: 6 in, 1 out]
          n233 = Build Array(w602, w601) -> (w603:dbl[])
          n234 = Add(x=w600, y=60.0) -> (x+y=w604:dbl)
        }
        n235 = for {
          N: 5 -> [_]
          shift-right: [w555] -> _
          shift-left: w479 -> [w558]
          tunnel: [w555] -> w478 mode=concatenating
          i -> [w554]
          n236 = for {
            tunnel: w558 -> [w589] mode=indexing
            tunnel: [w588] -> w556 mode=indexing
            n237 = in-place {
              n238 = in-place-array #3(w589, 0, 1) -> (w593:dbl, w592:dbl)
              n239 = Re/Im To Polar(2:w592, 3:w593) -> (0:w594:dbl, 1:w596:dbl)
              n240 = Add(x=w596, y=15.0) -> (x+y=w595:dbl)
              n241 = Polar To Re/Im(2:w594, 3:w595) -> (0:w590:dbl, 1:w591:dbl)
              n242 = in-place-array #3(w591, w590) -> (w588:dbl[])  [unwired: 2 out]
            }
          }
          n243 = Equal?(x=w554, y=4) -> (x = y?=w557:bool)
          n244 = case shown="True" w557 {
            tunnel: w556 -> [w559 w583]
            tunnel: [w559 w560] -> w555
            frame False {
            }
            frame True {
              n245 = Index Array(array=w583) -> (element #1=w562:dbl[], element #2=w580:dbl[], element #3=w575:dbl[], element #4=w571:dbl[], element #5=w567:dbl[], element #6=w563:dbl[])  [unwired: 12 in]
              n246 = Add(x=w562, y=w580) -> (x+y=w585:dbl[])
              n247 = Add(x=w580, y=w575) -> (x+y=w581:dbl[])
              n248 = Add(x=w575, y=w571) -> (x+y=w577:dbl[])
              n249 = Add(x=w563, y=w562) -> (x+y=w565:dbl[])
              n250 = Add(x=w571, y=w567) -> (x+y=w573:dbl[])
              n251 = Add(x=w567, y=w563) -> (x+y=w569:dbl[])
              n252 = Divide(x=w585, y=2.0) -> (x/y=w582:dbl[])
              n253 = Divide(x=w581, y=2.0) -> (x/y=w578:dbl[])
              n254 = Divide(x=w577, y=2.0) -> (x/y=w574:dbl[])
              n255 = Divide(x=w565, y=2.0) -> (x/y=w561:dbl[])
              n256 = Divide(x=w573, y=2.0) -> (x/y=w570:dbl[])
              n257 = Divide(x=w569, y=2.0) -> (x/y=w566:dbl[])
              n258 = Build Array (concatenate)(w583, w582, w578, w574, w570, w566, w561) -> (w560:dbl[][])
            }
          }
        }
        n259 = Build Array (concatenate)(w479, w478, dbl[] [0.0, 0.0] ("array")) -> (w476:dbl[][])
        n260 = for {
          tunnel: w476 -> [w548] mode=indexing
          tunnel: [w543] -> w474 mode=concatenating
          n261 = Index Array(array=w548) -> (element #1=w547:dbl, element #2=w546:dbl)  [unwired: 2 in]
          n262 = Build Array(5.0 ("element"), 1.0 ("element"), 0.0 ("element"), 0.0 ("element"), w547, w546, 0.0 ("element"), 0.0 ("element")) -> (w541:dbl[])
          n263 = Build Array(dbl[] [0.0, 0.0, 0.0, 0.0, 0.0, 0.0, 0.0, 0.0] ("array"), w541) -> (w543:dbl[][])
        }
        n264 = Build Array (concatenate)(w482, w474) -> (w473:dbl[][])
        n265 = for {
          tunnel: [w483] -> _ mode=indexing
          shift-right: [w484] -> w472
          shift-left: picture data[5B] ("new picture") -> [w485]
          tunnel: w473 -> [w483] mode=indexing
          n266 = Index Array(array=w483, index=0) -> (element=w486:dbl)
          n267 = case shown="7" w486 {
            tunnel: w483 -> [_ w505 w518 w536]
            tunnel: w485 -> [w488 w507 w520 w540]
            tunnel: [w488 w509 w519 w539] -> w484
            frame 0, Default {
            }
            frame 3 {
              w506 = TRUE ("absolute coordinates?(T)")
              n268 = Index Array(array=w505) -> (element #5=w500:dbl, element #6=w497:dbl, element #7=w499:dbl, element #8=w491:dbl)  [unwired: 8 in, 4 out]
              n269 = Negate(x=w500) -> (-x=w498:dbl)
              n270 = Negate(x=w499) -> (-x=w492:dbl)
              n271 = call-poly <vilib>:"2D Cartesian Coordinate Rotation.vi"("theta"=3.141592653589793, "y"=w497, "x"=w498) -> ("y out"=w494:dbl, "x out"=w495:dbl)  [unwired: 6 in, 1 out]
              n272 = call-poly <vilib>:"2D Cartesian Coordinate Rotation.vi"("theta"=3.141592653589793, "y"=w491, "x"=w492) -> ("y out"=w489:dbl, "x out"=w490:dbl)  [unwired: 6 in, 1 out]
              n273 = Build Array(w495, w494) -> (w504:dbl[])
              n274 = Build Array(w490, w489) -> (w502:dbl[])
              n275 = Array To Cluster(array=w504) -> (cluster=w503:cluster{"[0]":dbl, "[1]":dbl})
              n276 = Array To Cluster(array=w502) -> (cluster=w501:cluster{"[0]":dbl, "[1]":dbl})
              n277 = call <vilib>:"Move Pen.vi"("absolute coordinates?(T)"=w506, "new position"=w503, "picture"=w507) -> ("new picture"=w508:picture)  [unwired: 2 in]
              n278 = call <vilib>:"Draw Line.vi"("picture"=w508, "end point"=w501, "absolute coordinates?(T)"=w506) -> ("new picture"=w509:picture)  [unwired: 6 in]
            }
            frame 5 {
              n279 = Index Array(array=w518) -> (element #5=w515:dbl, element #6=w512:dbl)  [unwired: 6 in, 4 out]
              n280 = Negate(x=w515) -> (-x=w513:dbl)
              n281 = call-poly <vilib>:"2D Cartesian Coordinate Rotation.vi"("theta"=3.141592653589793, "y"=w512, "x"=w513) -> ("y out"=w510:dbl, "x out"=w511:dbl)  [unwired: 6 in, 1 out]
              n282 = Build Array(w511, w510) -> (w517:dbl[])
              n283 = Array To Cluster(array=w517) -> (cluster=w516:cluster{"[0]":dbl, "[1]":dbl})
              n284 = call <vilib>:"Draw Point.vi"("picture"=w520, "point(x,y)"=w516) -> ("new picture"=w519:picture)  [unwired: 7 in]
            }
            frame 7 {
              n285 = Index Array(array=w536) -> (element #3=w533:dbl, element #4=w528:dbl, element #5=w532:dbl, element #6=w523:dbl)  [unwired: 8 in, 4 out]
              n286 = Negate(x=w533) -> (-x=w529:dbl)
              n287 = Negate(x=w532) -> (-x=w526:dbl)
              n288 = call-poly <vilib>:"2D Cartesian Coordinate Rotation.vi"("theta"=3.141592653589793, "y"=w528, "x"=w529) -> ("y out"=w524:dbl, "x out"=w530:dbl)  [unwired: 6 in, 1 out]
              n289 = call-poly <vilib>:"2D Cartesian Coordinate Rotation.vi"("theta"=3.141592653589793, "y"=w523, "x"=w526) -> ("y out"=w522:dbl, "x out"=w525:dbl)  [unwired: 6 in, 1 out]
              n290 = Subtract(x=w525, y=w530) -> (x-y=w535:dbl)
              n291 = Subtract(x=w522, y=w524) -> (x-y=w521:dbl)
              n292 = Build Array(w530, w524) -> (w538:dbl[])
              n293 = Array To Cluster(array=w538) -> (cluster=w537:cluster{"[0]":dbl, "[1]":dbl})
              n294 = Re/Im To Polar(2:w521, 3:w535) -> (1:w534:dbl)  [unwired: 1 out]
              n295 = call <vilib>:"Draw Circle by Radius.vi"("pixel center"=w537, "radius"=w534, "picture"=w540) -> ("new picture"=w539:picture)  [unwired: 8 in]
            }
          }
        }
      }
    }
    "Array" <- w4
    "2D Picture" <- w5
  }
